vi "Controller - State Process.vi"(8 "error in (no error)":errorcluster, 11 "View Model":T1) -> (0 "error out":errorcluster, 3 "View Model":T1)   [LabVIEW 2017]
doc: "Processing the current state of Elevator controller."
uses:
  View Model/Controls/View Model.ctl
  View Model/Controls/Shared Model.ctl
  Error/Controls/Error Model.ctl
  Error/Controls/Error Event.ctl
  Error/Controls/Error Type.ctl
  Configuration/Controls/Config DB Model.ctl
  Configuration/Controls/Config DB Command.ctl
  Configuration/Controls/Config DB Record.ctl
  Controls/Controller Model.ctl
  Controls/Elevator Location.ctl
  Controls/Elevator Direction Event.ctl
  Controls/Elevator Direction.ctl
  Controls/Elevator CMD Event.ctl
  Controls/Elevator Commands.ctl
  Controls/Elevator Overhead.ctl
  Controls/Elevator State.ctl
  Controls/Elevator CMD Timer.ctl
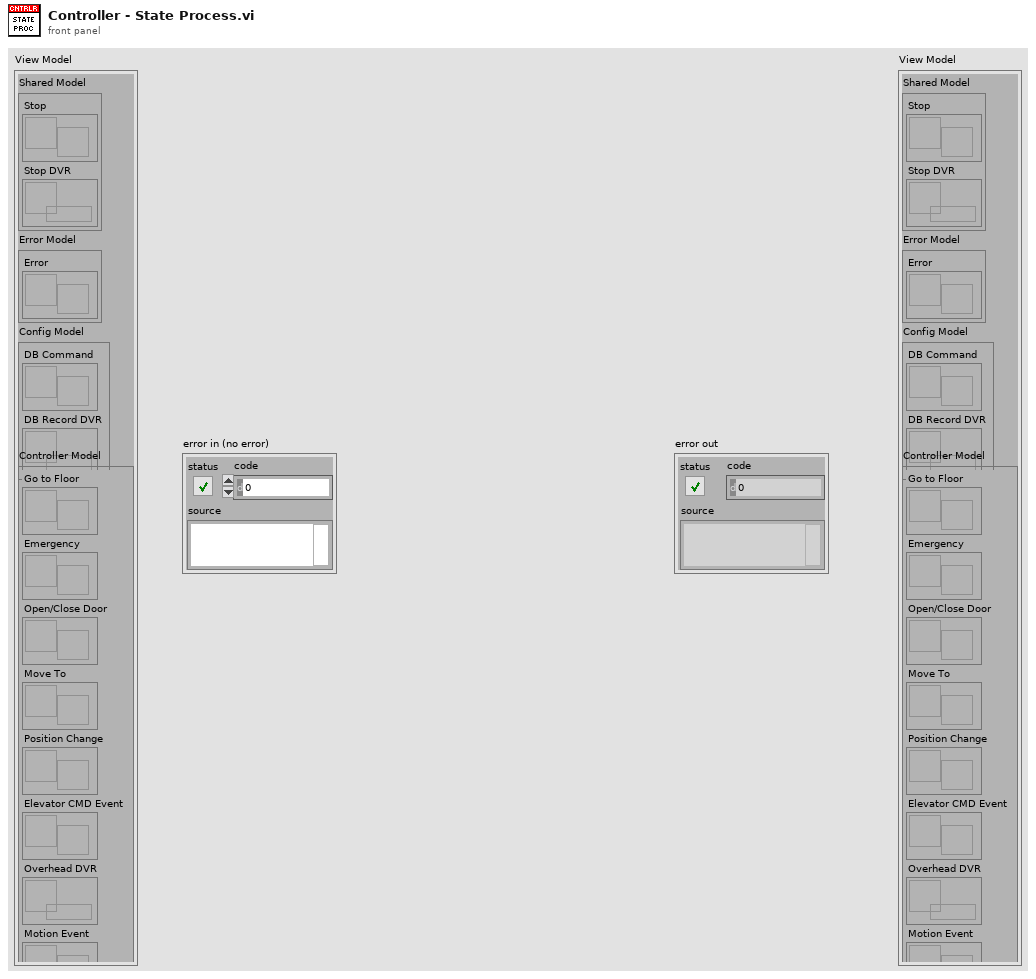
[diagram p1: front panel]
types:
  T1 = typedef "View Model.ctl" = cluster{"Shared Model":T2, "Error Model":T3, "Config Model":T4, "Controller Model":T5}
  T2 = typedef "Shared Model.ctl" = cluster{"Stop":refnum<user-event>, "Stop DVR":refnum<data-value>}
  T3 = typedef "Error Model.ctl" = cluster{"Error":refnum<user-event>}
  T4 = typedef "Config DB Model.ctl" = cluster{"DB Command":refnum<user-event>, "DB Record DVR":refnum<data-value>}
  T5 = typedef "Controller Model.ctl" = cluster{"Go to Floor":refnum<user-event>, "Emergency":refnum<user-event>, "Open/Close Door":refnum<user-event>, "Move To":refnum<user-event>, "Position Change":refnum<user-event>, "Elevator CMD Event":refnum<user-event>, "Overhead DVR":refnum<data-value>, "Motion Event":refnum<user-event>}
  T6 = typedef "Elevator State.ctl" = enum16{"No Request", "Initial", "Wait for 1st Request", "Start and Move", "Analysis", "Continue Travel", "Stop at Floor", "Open/Close Door", "Emergency", "Terminate"}
  T7 = typedef "Elevator CMD Timer.ctl" = enum16{"Start", "Get Time", "Pause", "Unpause"}
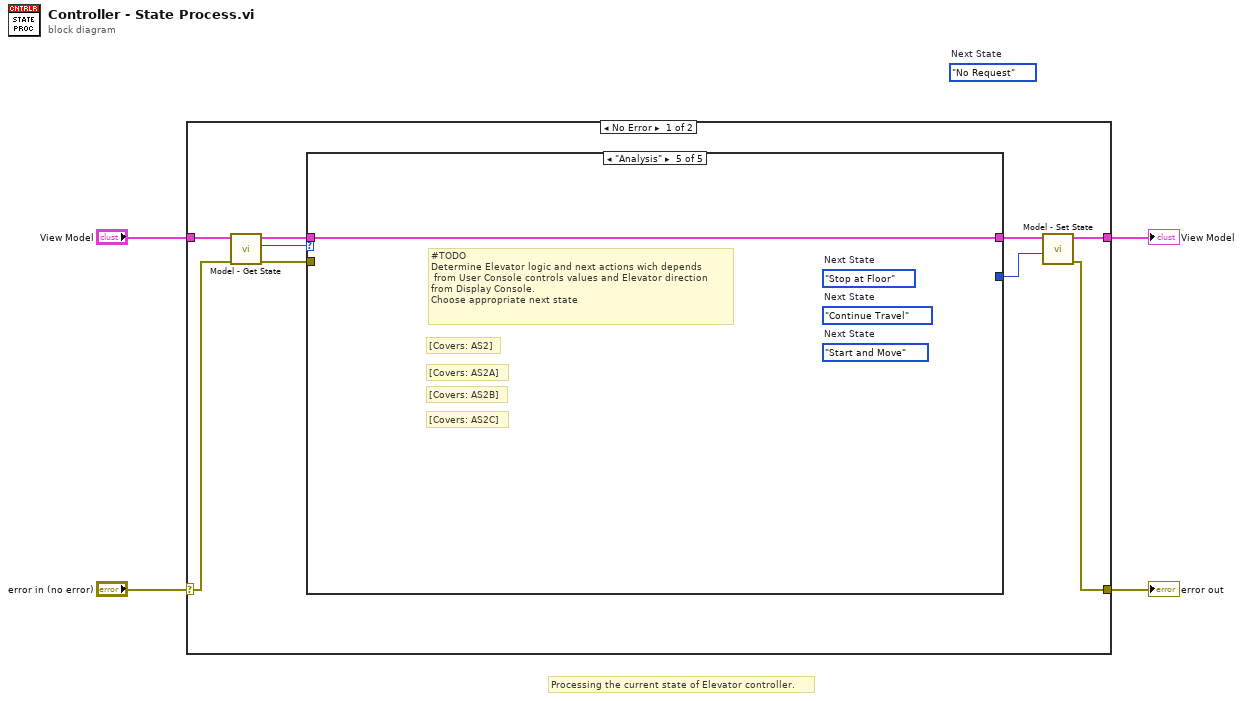
[diagram p0: block diagram]
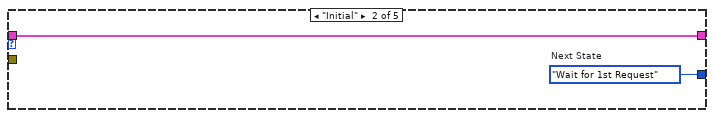
[diagram p3: hidden frame]
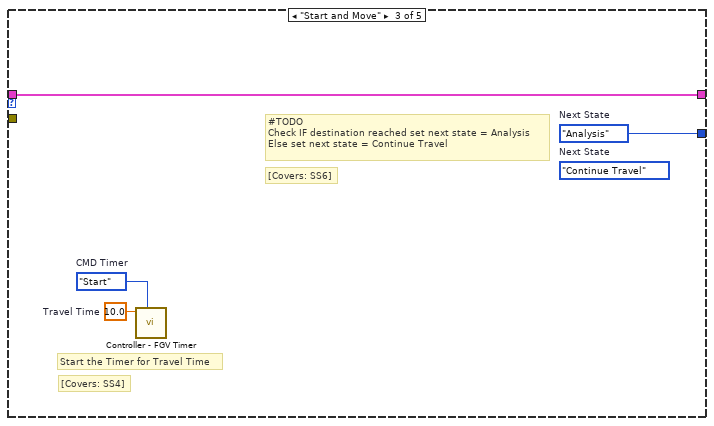
[diagram p4: hidden frame]
diagram:
  (unwired) Elevator_State."No Request"  # Next State
  # "Processing the current state of Elevator controller."
  n1 = case shown="No Error" "error in (no error)" {
    selector: "error in (no error)" -> [w12 w23]
    tunnel: "View Model" -> [w13 w24]
    tunnel: [w8 w24] -> w2
    tunnel: [w7 w23] -> w1
    frame No Error {
      n2 = call "Model - Get State.vi"("error in (no error)"=w12, "View Model"=w13) -> ("error out"=w10:errorcluster, "Current State"=w11:T6, "View Model"=w9:T1)  [unwired: 6 in, 1 out]
      n3 = case shown="\"Analysis\"" w11 {
        tunnel: w10 -> [_ _ _ _ _]
        tunnel: w9 -> [w14 w16 w20 w21 w22]
        tunnel: [w14 w16 w20 w21 w22] -> w6
        tunnel: [_ w15 w17 _ _] -> w5
        frame "No Request", Default {
        }
        frame "Initial" {
          w15 = Elevator_State."Wait for 1st Request"  # Next State
        }
        frame "Start and Move" {
          w17 = Elevator_State."Analysis"  # Next State
          (unwired) Elevator_State."Continue Travel"  # Next State
          w18 = 10.0  # Travel Time
          w19 = Elevator_CMD_Timer."Start"  # CMD Timer
          # "[Covers: SS6]"
          # "#TODO\nCheck IF destination reached set next state = Analysis\nElse set next state = Continue Travel"
          # "[Covers: SS4]"
          # "Start the Timer for Travel Time"
          n4 = call "Controller - FGV Timer.vi"("CMD Timer"=w19, "Target Time"=w18) -> ()  [unwired: 7 in, 3 out]
        }
        frame "Open/Close Door" {
          # "[Covers: SS1]"
          # "#TODO\nComplete Open/Close Door sequence\nand set nex state Start and Move"
        }
        frame "Analysis" {
          (unwired) Elevator_State."Start and Move"  # Next State
          (unwired) Elevator_State."Continue Travel"  # Next State
          (unwired) Elevator_State."Stop at Floor"  # Next State
          # "[Covers: AS2C]"
          # "[Covers: AS2B]"
          # "[Covers: AS2A]"
          # "[Covers: AS2]"
          # "#TODO\nDetermine Elevator logic and next actions wich depends\n from User Console controls values and Elevator direction\nfrom Display Console.\nChoose appropriate next state"
        }
      }
      n5 = call "Model - Set State.vi"("Next State"=w5, "View Model"=w6) -> ("error out"=w7:errorcluster, "View Model"=w8:T1)  [unwired: 8 in]
    }
    frame Error {
    }
  }
  "error out" <- w1
  "View Model" <- w2
